vi "Make_data_file.vi"(1 "File Name":string) -> (0 "File Refnum":refnum<file>)   [LabVIEW 2016]
panel:
  in  "dup path":path
  in  "Error In":errorcluster
  out "Error Out":errorcluster
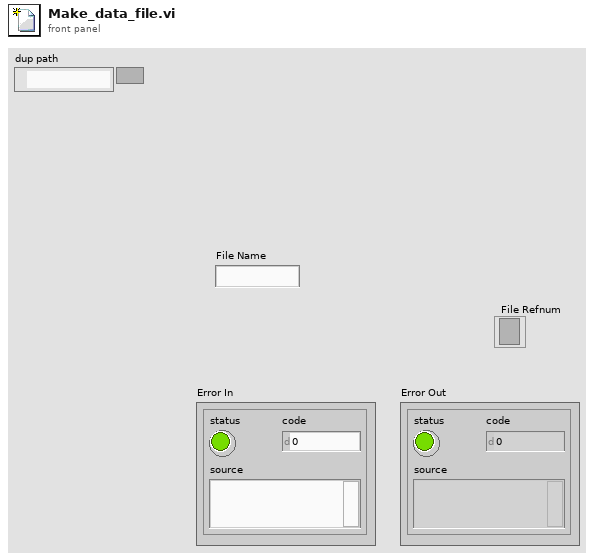
[diagram p1: front panel]
types:
  T1 = enum16{"open", "replace", "create", "open or create", "replace or create", "replace or create with confirmation"}
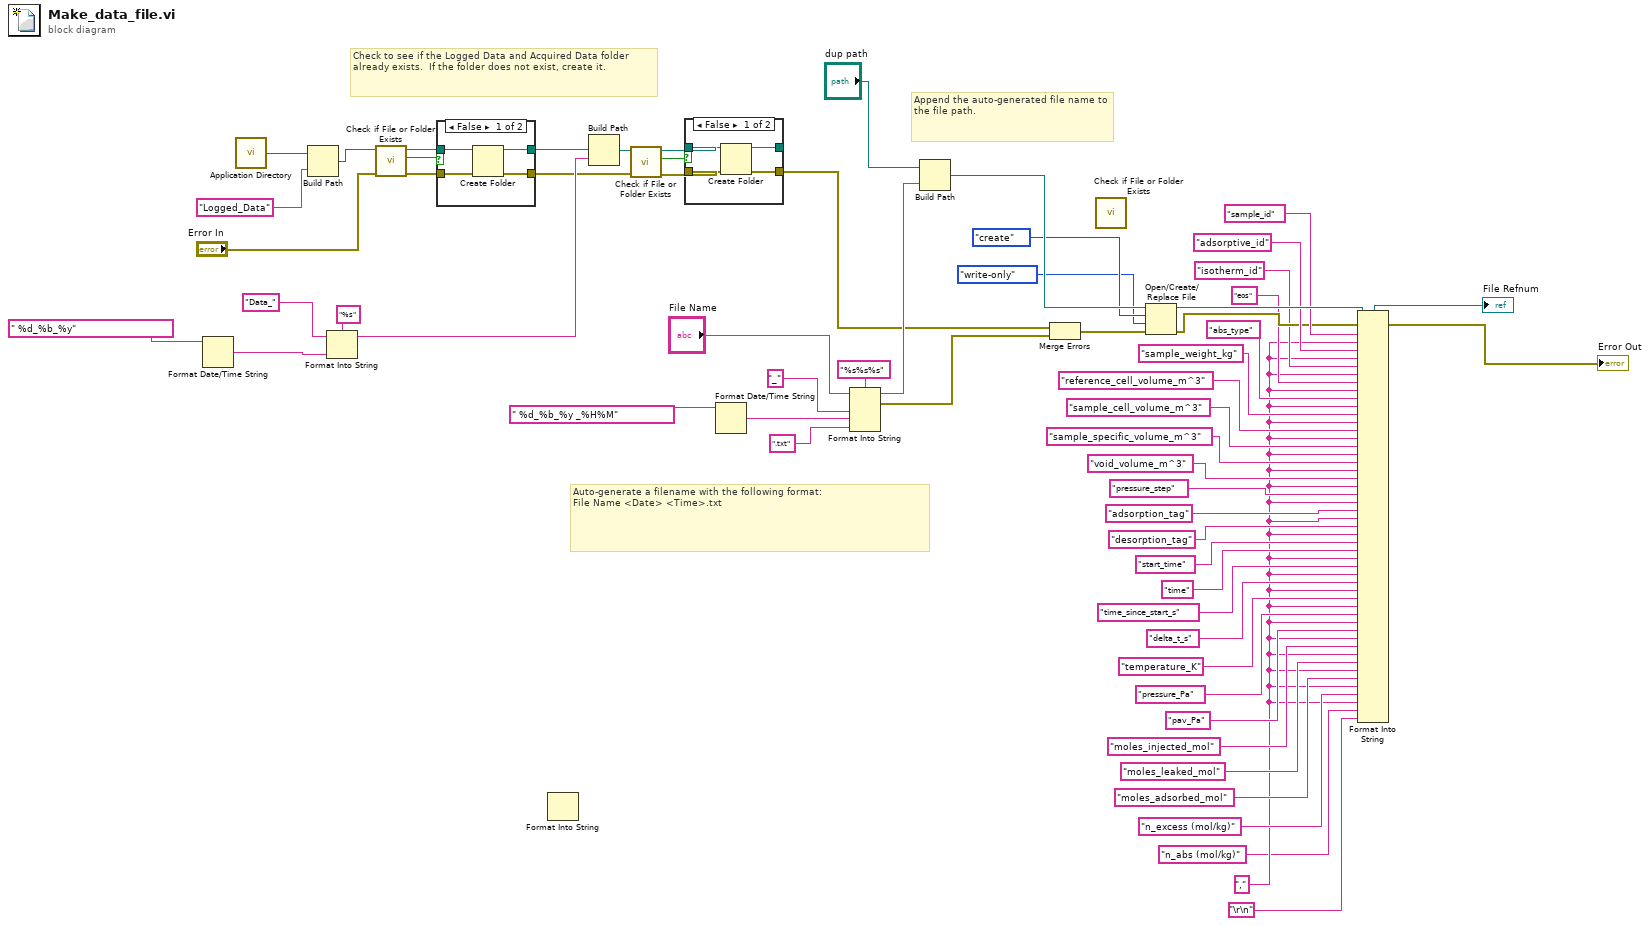
[diagram p0: block diagram]
diagram:
  w3 = "," ("input 2")
  # "Append the auto-generated file name to the file path."
  # "Check to see if the Logged Data and Acquired Data folder already exists.  If the folder does not exist, create it."
  # "Auto-generate a filename with the following format:\nFile Name <Date> <Time>.txt"
  n1 = Format Date/Time String(time format string (%c)=" %d_%b_%y") -> (date/time string=w45:string)  [unwired: 2 in]
  n2 = call <vilib>:"Application Directory.vi"() -> ("Application Directory"=w53:path)
  n3 = Build Path(base path=w53, name or relative path="Logged_Data" ("prompt (Create Folder)")) -> (appended path=w57:path)
  n4 = Format Into String(format string="%s", initial string="Data_" ("string"), w45) -> (resulting string=w43:string)  [unwired: 1 in, 1 out]
  n5 = call <vilib>:"Check if File or Folder Exists.vi"("error in (no error)"="Error In", "path"=w57) -> ("error out"=w56:errorcluster, "file or folder exists?"=w54:bool, "dup path"=w55:path)  [unwired: 7 in]
  n6 = case shown="False" w54 {
    tunnel: [w67 w69] -> w48
    tunnel: [w66 w68] -> w42
    tunnel: w56 -> [w65 w68]
    tunnel: w55 -> [w64 w69]
    frame False {
      n7 = Create Folder(path (use dialog)=w64, error in=w65) -> (created path=w67:path, error out=w66:errorcluster)  [unwired: 1 in, 1 out]
    }
    frame True {
    }
  }
  n8 = Format Into String() -> ()  [unwired: 4 in, 2 out]
  n9 = Build Path(base path=w48, name or relative path=w43) -> (appended path=w41:path)
  n10 = call <vilib>:"Check if File or Folder Exists.vi"("error in (no error)"=w42, "path"=w41) -> ("error out"=w38:errorcluster, "file or folder exists?"=w39:bool, "dup path"=w40:path)  [unwired: 7 in]
  n11 = case shown="False" w39 {
    tunnel: [w73 w75] -> _
    tunnel: [w72 w74] -> w37
    tunnel: w38 -> [w71 w74]
    tunnel: w40 -> [w70 w75]
    frame False {
      n12 = Create Folder(path (use dialog)=w70, error in=w71) -> (created path=w73:path, error out=w72:errorcluster)  [unwired: 1 in, 1 out]
    }
    frame True {
    }
  }
  n13 = Format Date/Time String(time format string (%c)=" %d_%b_%y _%H%M") -> (date/time string=w35:string)  [unwired: 2 in]
  n14 = Format Into String(format string="%s%s%s", initial string="File Name", "_" ("input 1"), w35, ".txt" ("string")) -> (resulting string=w49:string, error out=w50:errorcluster)  [unwired: 1 in]
  n15 = Build Path(base path="dup path", name or relative path=w49) -> (appended path=w63:path)
  n16 = Merge Errors(w37, w50) -> (w62:errorcluster)
  n17 = call <vilib>:"Check if File or Folder Exists.vi"() -> ()  [unwired: 9 in, 3 out]
  n18 = Open/Create/Replace File(file path (use dialog)=w63, error in=w62, operation (0:open)=T1."create", access (0:read/write)=enum16{"read/write", "read-only", "write-only"}."write-only") -> (refnum out=w32:refnum<file>, error out=w28:errorcluster)  [unwired: 2 in, 1 out]
  n19 = Format Into String(initial string=w32, error in=w28, "sample_id", w3, "adsorptive_id", w3, "isotherm_id" ("input 5"), w3, "eos" ("input 7"), w3, "abs_type" ("input 9"), w3, "sample_weight_kg" ("input 11"), w3, "reference_cell_volume_m^3", w3, "sample_cell_volume_m^3", w3, "sample_specific_volume_m^3", w3, "void_volume_m^3", w3, "pressure_step", w3, "adsorption_tag", w3, "desorption_tag", w3, "start_time", "time", w3, "time_since_start_s", w3, "delta_t_s", w3, "temperature_K", w3, "pressure_Pa", w3, "pav_Pa", w3, "moles_injected_mol", w3, "moles_leaked_mol", w3, "moles_adsorbed_mol", w3, "n_excess (mol/kg)", w3, "n_abs (mol/kg)" ("input 7"), "\r\n") -> (resulting string=→"File Refnum":refnum<file>, error out=→"Error Out":errorcluster)  [unwired: 1 in]
